vi "Get Installed Fonts.vi"(8 "Error In":errorcluster) -> (0 "Error Out":errorcluster, 1 "# Fonts":i32, 3 "Installed Fonts":string[](array[string]))   [LabVIEW 2021, in "Rich Text Box.lvlib"]
uses:
  System.Drawing
  Rich Text Box.lvlib
panel:
  # "see the License on the block diagram (Ctrl+E or Window:Show Block Diagram)"
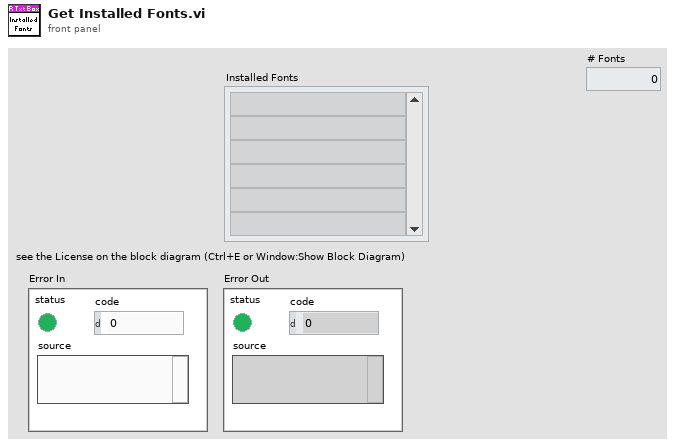
[diagram p1: front panel]
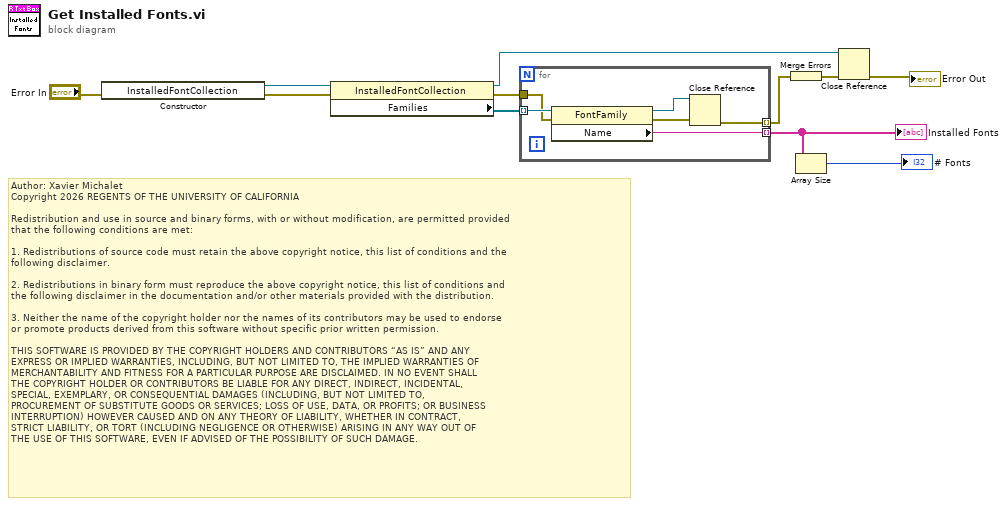
[diagram p0: block diagram]
diagram:
  # "Author: Xavier Michalet\nCopyright 2026 REGENTS OF THE UNIVERSITY OF CALIFORNIA\n\nRedistribution and use in source and binary forms, with or without modification, are permitted provided\nthat the following conditions are met:\n\n1. Redistributions of source code must retain the above copyright notice, this list of conditions and the\nfollowing disclaimer.\n\n2. Redistributions in binary form must reproduce the above copyright notice, this list of conditions and\nthe following disclaimer in the documentation and/or other materials provided with the distribution.\n\n3. Neither the name of the copyright holder nor the names of its contributors may be used to endorse \nor promote products derived from this software without specific prior written permission.\n\nTHIS SOFTWARE IS PROVIDED BY THE COPYRIGHT HOLDERS AND CONTRIBUTORS “AS IS” AND ANY \nEXPRESS OR IMPLIED WARRANTIES, INCLUDING, BUT NOT LIMITED TO, THE IMPLIED WARRANTIES OF\nMERCHANTABILITY AND FITNESS FOR A PARTICULAR PURPOSE ARE DISCLAIMED. IN NO EVENT SHALL\nTHE COPYRIGHT HOLDER OR CONTRIBUTORS BE LIABLE FOR ANY DIRECT, INDIRECT, INCIDENTAL, \nSPECIAL, EXEMPLARY, OR CONSEQUENTIAL DAMAGES (INCLUDING, BUT NOT LIMITED TO, \nPROCUREMENT OF SUBSTITUTE GOODS OR SERVICES; LOSS OF USE, DATA, OR PROFITS; OR BUSINESS\nINTERRUPTION) HOWEVER CAUSED AND ON ANY THEORY OF LIABILITY, WHETHER IN CONTRACT, \nSTRICT LIABILITY, OR TORT (INCLUDING NEGLIGENCE OR OTHERWISE) ARISING IN ANY WAY OUT OF\nTHE USE OF THIS SOFTWARE, EVEN IF ADVISED OF THE POSSIBILITY OF SUCH DAMAGE."
  n1 = constructor class="InstalledFontCollection"(error in="Error In") -> (reference out=w11:refnum<k24>, error out=w9:errorcluster)  [unwired: 2 in, 1 out]
  n2 = property class="InstalledFontCollection"(reference=w11, error in=w9) -> (reference out=w7:refnum<k24>, error out=w8:errorcluster, "Families"=w10:refnum<k24>[])
  n3 = for {
    tunnel: w10 -> [w16] mode=indexing
    tunnel: [w17] -> w4 mode=indexing
    tunnel: w8 -> [w13]
    tunnel: [w12] -> w6 mode=indexing
    n4 = property class="FontFamily"(reference=w16, error in=w13) -> (reference out=w14:refnum<k24>, error out=w15:errorcluster, "Name"=w17:string)
    n5 = Close Reference(reference=w14, error in (no error)=w15) -> (error out=w12:errorcluster)
  }
  "Installed Fonts" <- w4
  n6 = Merge Errors(w6) -> (w5:errorcluster)
  n7 = Array Size(array=w4) -> (size(s)=→"# Fonts":i32)
  n8 = Close Reference(reference=w7, error in (no error)=w5) -> (error out=→"Error Out":errorcluster)
